vi "Add RX Packet to Stats.vi"(7 "Packet":T1, 8 "error in (no error)":errorcluster, 11 "Name":string) -> (0 "error out":errorcluster)   [LabVIEW 2023, in "WebSocket.lvclass"]
uses:
  WebSocket.lvclass
  WebSocket Packet.ctl
  private/Fixed Header.ctl
  private/OpCode.ctl
  WebSocket Stats VIG Mode.ctl
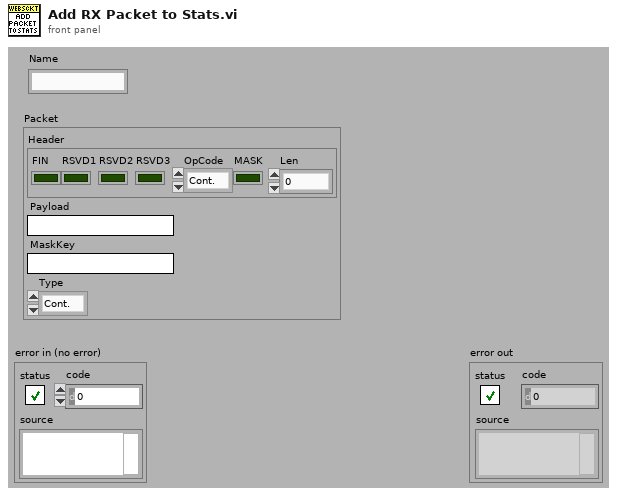
[diagram p1: front panel]
types:
  T1 = typedef "WebSocket.lvclass/WebSocket Packet.ctl" = cluster{"Header":T2, "Payload":string, "MaskKey":string, "Type":T3}
  T2 = typedef "WebSocket.lvclass/Fixed Header.ctl" = cluster{"FIN":bool, "RSVD1":bool, "RSVD2":bool, "RSVD3":bool, "OpCode":T3, "MASK":bool, "Len":u8}
  T3 = typedef "WebSocket.lvclass/OpCode.ctl" = enum16{"Cont.", "Text", "Binary", "NonCtl3", "NonCtl4", "NonCtl5", "NonCtl6", "NonCtl7", "Close", "Ping", "Pong", "Rsvd11", "Rsvd12", "Rsvd13", "Rsvd14", "Rsvd15"}
  T4 = typedef "WebSocket Stats VIG Mode.ctl" = enum16{"Init", "Set", "Update", "Get All"}
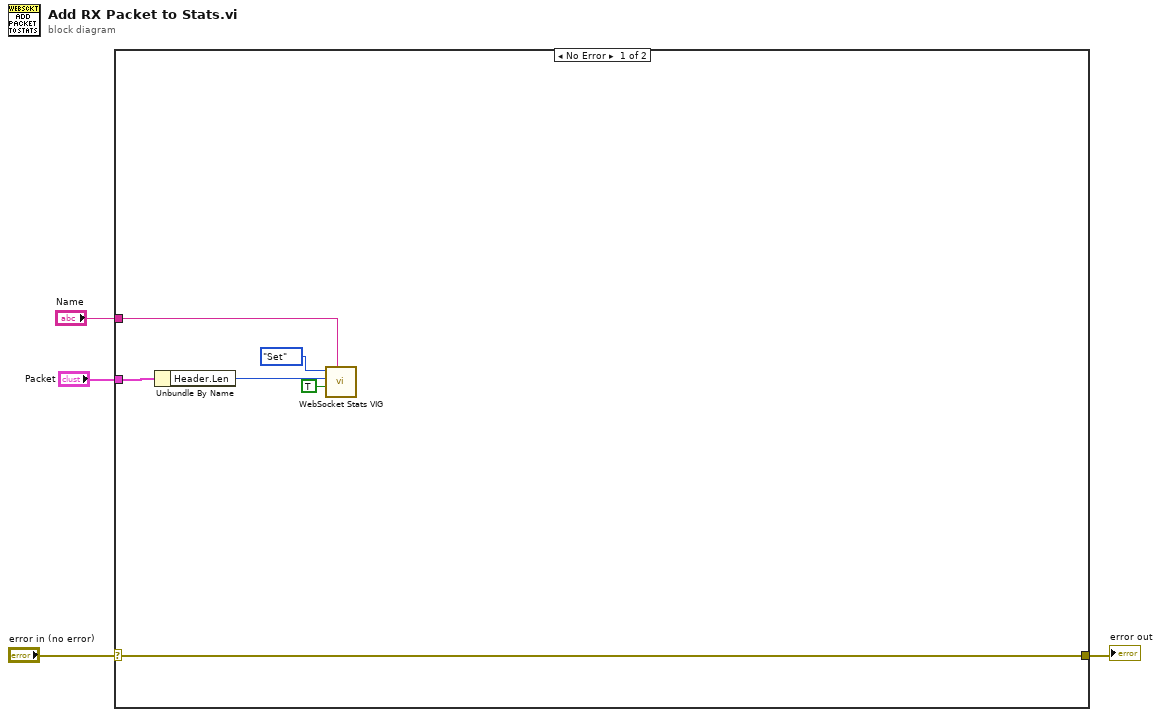
[diagram p0: block diagram]
diagram:
  n1 = case shown="No Error" "error in (no error)" {
    selector: "error in (no error)" -> [w9 w11]
    tunnel: [w9 w11] -> w3
    tunnel: "Packet" -> [w10 _]
    tunnel: "Name" -> [w6 _]
    frame No Error {
      n2 = Unbundle By Name(w10) -> ("Header.Len"=w8:u8)
      n3 = call "WebSocket Stats VIG.vi"("Name"=w6, "RX?"=TRUE, "Length"=w8, "mode"=WebSocket_Stats_VIG_Mode."Set") -> ()  [unwired: 5 in, 3 out]
    }
    frame Error {
    }
  }
  "error out" <- w3
